vi "C8855-01_WriteToSpreadsheetFile.vi"(0 "delimiter (Tab)":string="\t" caption="デリメタ(タブ)", 4 "transpose? (no:F)":bool caption="転置? (しない:F)", 5 "format (%.3f)":string="%.3f" caption="形式 (%.3f)", 6 "pattern":string="*.xls" caption="パターン", 8 "append to file? (new file:F)":bool caption="ファイルに連結? (新規ファイル:F)", 9 "1D data":sgl[](array[numeric]) caption="1次元データ" format="%.2f", 10 "2D data":sgl[][](array[numeric]) caption="2次元データ" format="%.2f", 11 "file path (dialog if empty)":path caption="ファイルパス (空の場合、ダイアログ)") -> (3 "new file path (Not A Path if cancelled)":path caption="新規ファイルパス（キャンセルされた場合はパスではない）")   [LabVIEW 2017]
doc: "単精度(SGL)数値の2次元または1次元配列をテキスト文字列に変換し、その文字列を新規バイトストリームファイルに書き込むか、または既存のファイルに追加します。"
panel:
  in  "prompt":string="書き込むファイルを選択。" caption="プロンプト"
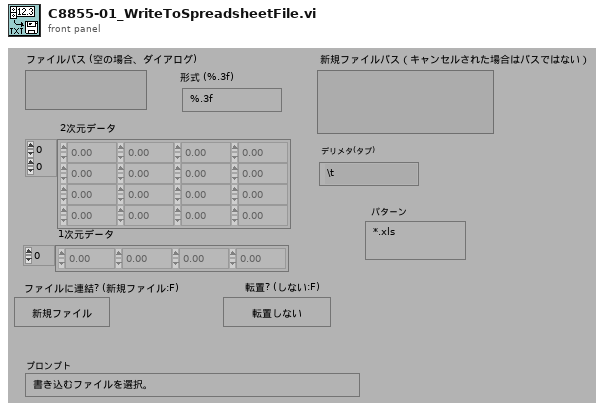
[diagram p1: front panel]
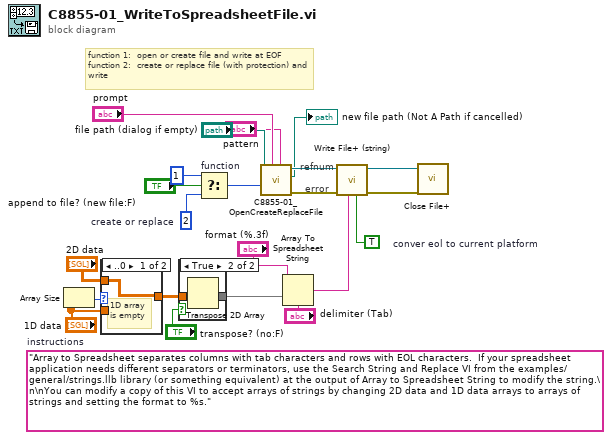
[diagram p0: block diagram]
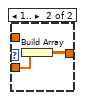
[diagram p3: hidden frame]
diagram:
  (unwired) "Array to Spreadsheet separates columns with tab characters and rows with EOL characters.  If your spreadsheet application needs different separators or terminators, use the Search String and Replace VI from the examples/general/strings.llb library (or something equivalent) at the output of Array to Spreadsheet String to modify the string.\n\nYou can modify a copy of this VI to accept arrays of strings by changing 2D data and 1D data arrays to arrays of strings and setting the format to %s."  # instructions
  w4 = i16 2  # create or replace
  w10 = TRUE  # conver eol to current platform
  # "error"
  # "refnum"
  # "function 1:  open or create file and write at EOF\nfunction 2:  create or replace file (with protection) and write"
  n1 = Array Size(array="1D data") -> (size(s)=w21:i32)
  n2 = case shown="..0" w21 {
    tunnel: "1D data" -> [_ w25]
    tunnel: [w23 w24] -> w17
    tunnel: "2D data" -> [w23 _]
    frame ..0 {
      # "1D array is empty"
    }
    frame 1.. {
      n3 = Build Array(w25) -> (w24:sgl[][])
    }
  }
  n4 = case shown="TRUE" "transpose? (no:F)" {
    tunnel: [w26 w28] -> w15
    tunnel: w17 -> [w26 w27]
    frame False {
    }
    frame True {
      n5 = Transpose 2D Array(2D array=w27) -> (transposed array=w28:sgl[][])
    }
  }
  n6 = Select "function"(t=i16 1, s="append to file? (new file:F)", f=w4) -> (s? t:f=w5:i16)
  n7 = call "C8855-01_OpenCreateReplaceFile.vi"("pattern"="pattern", "prompt"="prompt", "function (open:0)"=w5, "file path"="file path (dialog if empty)") -> ("error out"=w13:errorcluster, "new file path"=→"new file path (Not A Path if cancelled)":path, "refnum"=w9:refnum<file>)  [unwired: 3 in, 2 out]
  n8 = Array To Spreadsheet String(delimiter (Tab)="delimiter (Tab)", array=w15, 3:"format (%.3f)") -> (spreadsheet string=w12:string)
  n9 = call <vilib>:"Write File+ (string).vi"("convert eol? (no:F)"=w10, "string"=w12, "error in (no error)"=w13, "refnum"=w9) -> ("error out"=w22:errorcluster, "dup refnum"=w11:refnum<file>)  [unwired: 2 in, 2 out]
  n10 = call <vilib>:"Close File+.vi"("error in (no error)"=w22, "refnum"=w11) -> ()  [unwired: 6 out]
